vi "LSX Stop Axes Ex.vi"(8 "error in (no error)":errorcluster, 10 "lFlags":i32, 11 "lLSID":i32) -> (0 "error out":errorcluster, 3 "function return":i32)   [LabVIEW 2016, in "Tango_DLL.lvlib"]
doc: "TANGOAPI int TANGOCALL LSX_StopAxesEx (int lLSID, int lFlags);"
uses:
  Tango_DLL.lvlib
  2017/Microscope Control/Device Library/Stages/Marzhauser/SCAN IM 120 x 80/Tango DLL VIs/Tango_DLL.dll
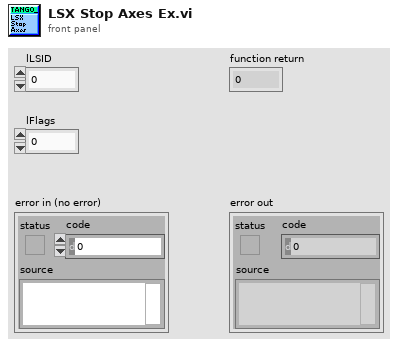
[diagram p1: front panel]
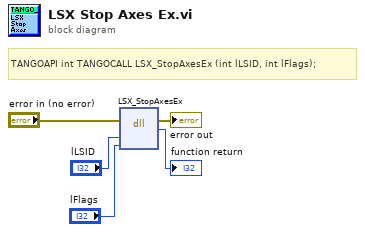
[diagram p0: block diagram]
diagram:
  # "TANGOAPI int TANGOCALL LSX_StopAxesEx (int lLSID, int lFlags);"
  n1 = dll-call lib="C:/Users/4PiSMS/Documents/Microscope Control/2017/Microscope Control/Device Library/Stages/Marzhauser/SCAN IM 120 x 80/Tango DLL VIs/Tango_DLL.*" fn="LSX_StopAxesEx"(error in="error in (no error)", "lLSID"="lLSID", "lFlags"="lFlags") -> (error out=→"error out":errorcluster, →"function return":i32)  [unwired: 4 in, 1 out]
